vi "Initialise.vi"(8 "error in":errorcluster, 9 "Radial Points":i32) -> (0 "error out":errorcluster, 3 "Model Data":T2 {"Matricies"."K" format="%#_6e"; "Matricies"."Dout" format="%#_6e"; "Matricies"."Bout" format="%#_6e"; "Matricies"."Aout" format="%#_6e"; "Matricies"."Dint" format="%#_6e"; "Matricies"."Bint" format="%#_6e"; "Matricies"."Aint" format="%#_6e"; "Constants"."Z" format="%^#_6e"})   [LabVIEW 2012]
uses:
  Model Data.ctl
  PZT type.ctl
  Piezo_Discs.ctl
  LEM_Params.ctl
  Layer Properties.ctl
  Matricies.ctl
  <vilib>/Utility/error.llb/DialogType.ctl
  <vilib>/Analysis/1siggen.llb/Ramp Pattern by Samples.vi
  <vilib>/Analysis/NI_AALBase.lvlib
panel:
  out "Layer Properties":T1[](array[typedef])
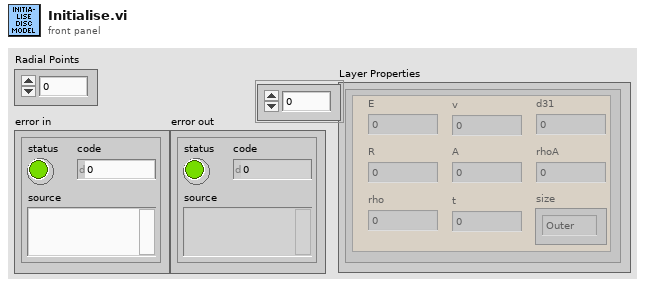
[diagram p1: front panel]
types:
  T1 = typedef "Layer Properties.ctl" = cluster{"E":dbl, "R":dbl, "rho":dbl, "rhoA":dbl, "v":dbl, "A":dbl, "t":dbl, "d31":dbl, "size":enum16{"Outer", "Inner"}}
  T2 = typedef "Model Data.ctl" = cluster{"Disc Properties":cluster{"Type":T3, "Disc Model":T4}, "Constants":cluster{"Radius":dbl[], "U(r)":dbl[], "W(r)":dbl[], "Vac":dbl, "P":dbl, "RiRo":dbl, "Area Density (r)":dbl[], "Ro":dbl, "Ri":dbl, "Z":dbl[], "Nr":dbl, "Mr":dbl, "c":dbl[], "AoC":dbl, "BoC":dbl, "AiC":dbl, "BiC":dbl, "f1":dbl, "f2":dbl}, "LEM Parameters":T5, "Layer Properties":T1[], "Matricies":T6}
  T3 = typedef "PZT type.ctl" = enum16{"Bimorph", "Unimorph"}
  T4 = typedef "Piezo_Discs.ctl" = enum16{"FTBD-21T-4.0A1", "PZT-5A (Gallas 1)", "PZT-5A (Gallas 2)", "AB4113B", "Create new disc...", "Load disc from file..."}
  T5 = typedef "LEM_Params.ctl" = cluster{"Displacement Ratio":dbl, "Cd":dbl, "Md":dbl, "xdc":dbl, "fd":dbl, "Sensitivity":dbl, "dA":dbl, "Rd":dbl, "Zeta":dbl, "Phi":dbl}
  T6 = typedef "Matricies.ctl" = cluster{"Aint":dbl[][], "Bint":dbl[][], "Dint":dbl[][], "Aout":dbl[][], "Bout":dbl[][], "Dout":dbl[][], "b":dbl[], "K":dbl[][]}
  T7 = typedef "DialogType.ctl" = u16
  T8 = typedef "Custom_Piezo.ctl" = cluster{"Young's Modulus":dbl, "Radius":dbl, "Density":dbl, "Poissoin's Ratio":dbl, "Thickness":dbl, "Dielectric Strength (d31)":dbl, "Type":T3}
  T9 = cluster{"Radius":dbl[], "U(r)":dbl[], "W(r)":dbl[], "Vac":dbl, "P":dbl, "RiRo":dbl, "Area Density (r)":dbl[], "Ro":dbl, "Ri":dbl, "Z":dbl[], "Nr":dbl, "Mr":dbl, "c":dbl[], "AoC":dbl, "BoC":dbl, "AiC":dbl, "BiC":dbl, "f1":dbl, "f2":dbl}
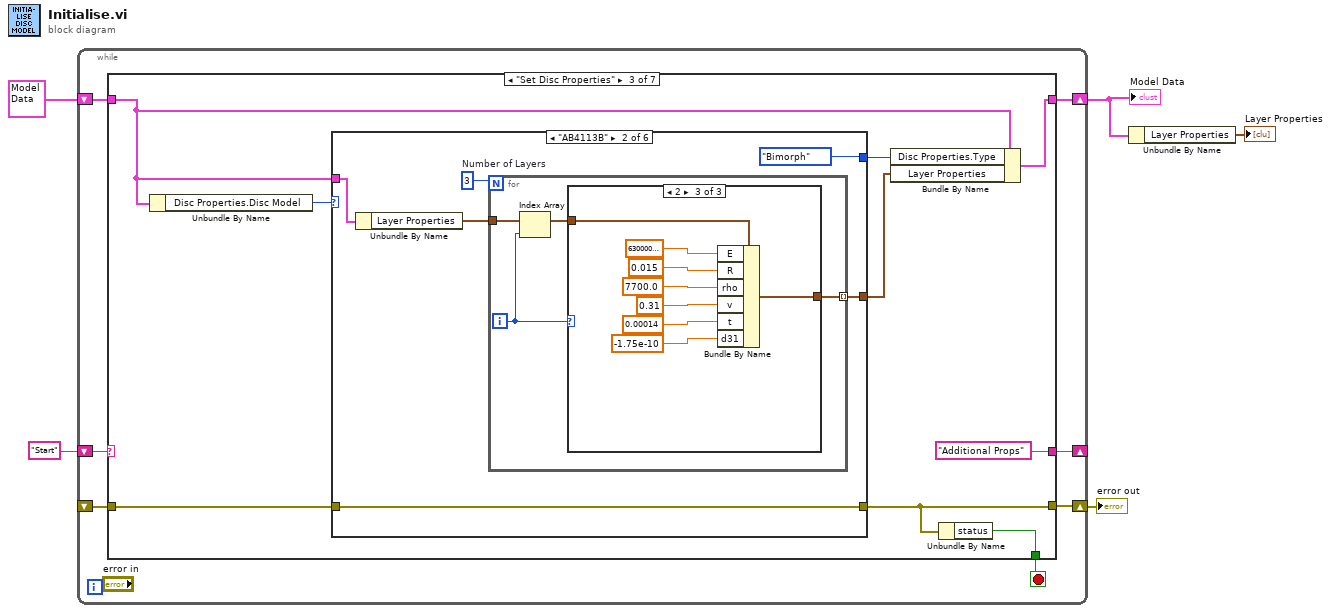
[diagram p0: block diagram]
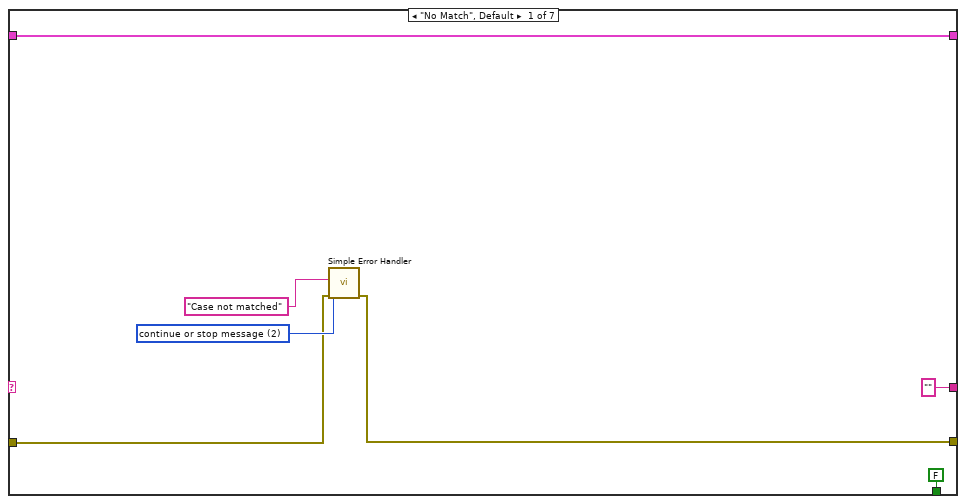
[diagram p2: hidden frame]
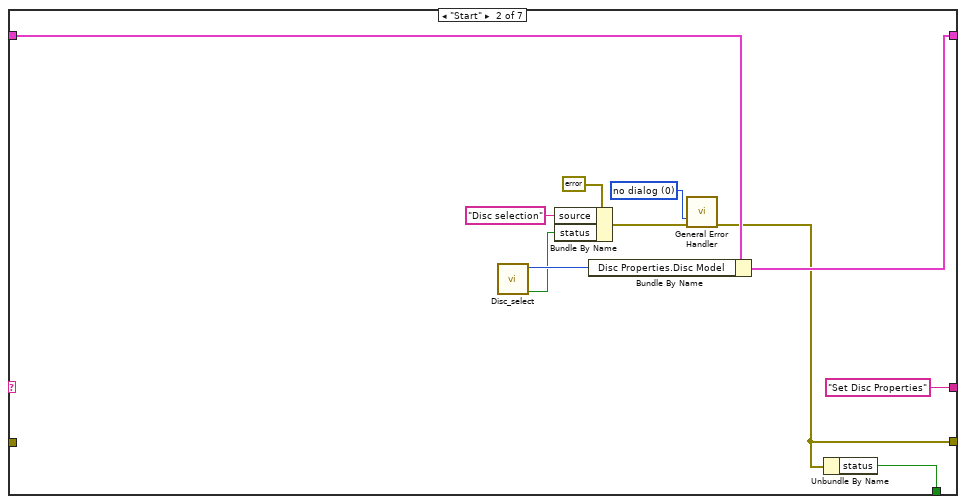
[diagram p3: hidden frame]
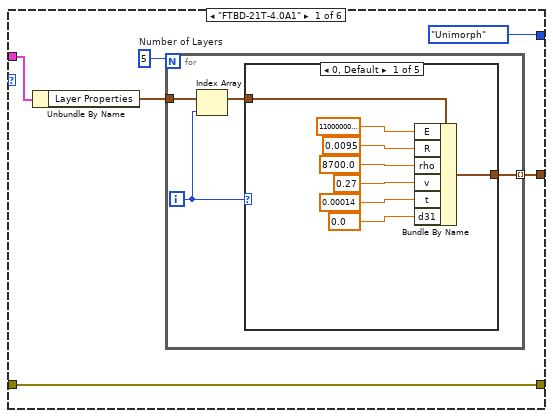
[diagram p4: hidden frame]
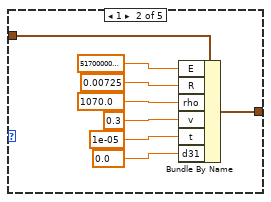
[diagram p5: hidden frame]
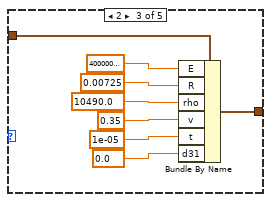
[diagram p6: hidden frame]
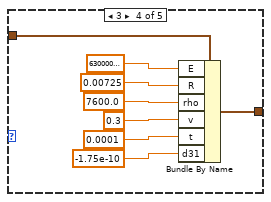
[diagram p7: hidden frame]
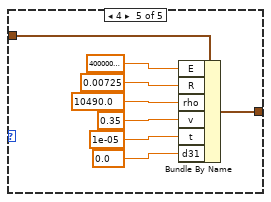
[diagram p8: hidden frame]
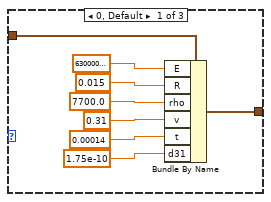
[diagram p9: hidden frame]
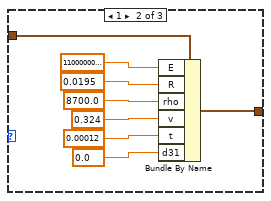
[diagram p10: hidden frame]
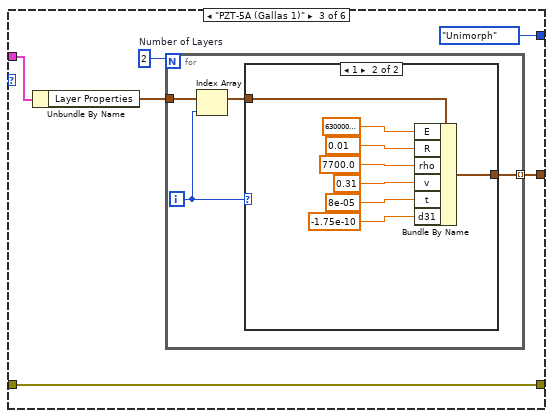
[diagram p11: hidden frame]
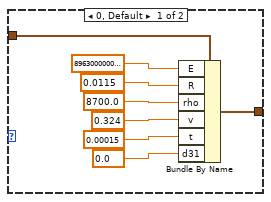
[diagram p12: hidden frame]
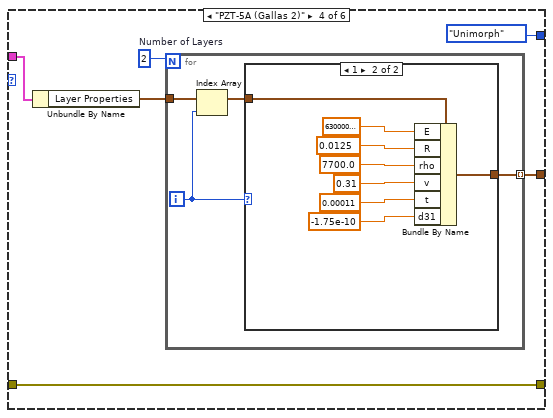
[diagram p13: hidden frame]
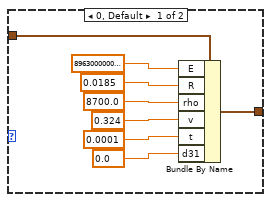
[diagram p14: hidden frame]
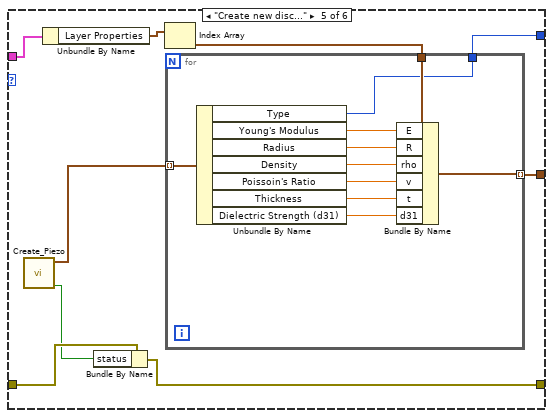
[diagram p15: hidden frame]
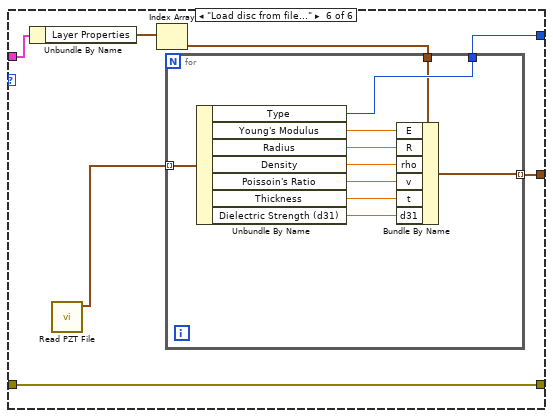
[diagram p16: hidden frame]
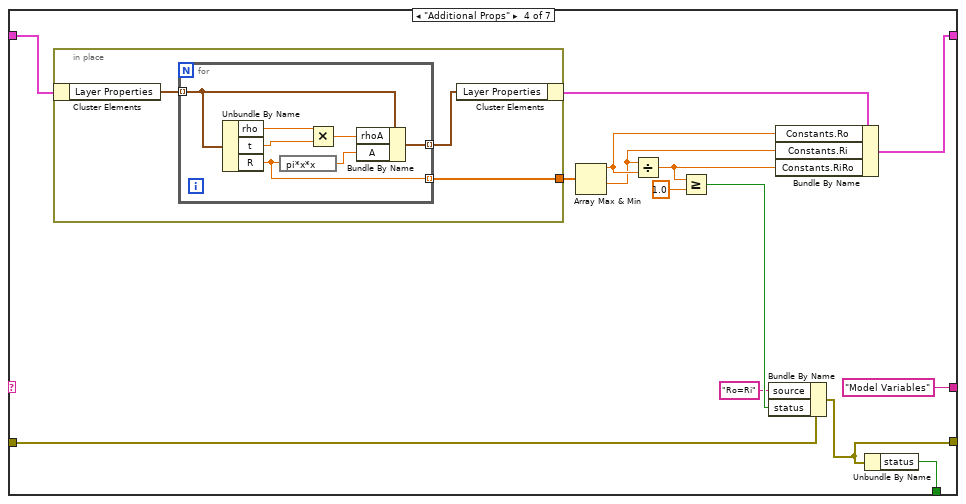
[diagram p17: hidden frame]
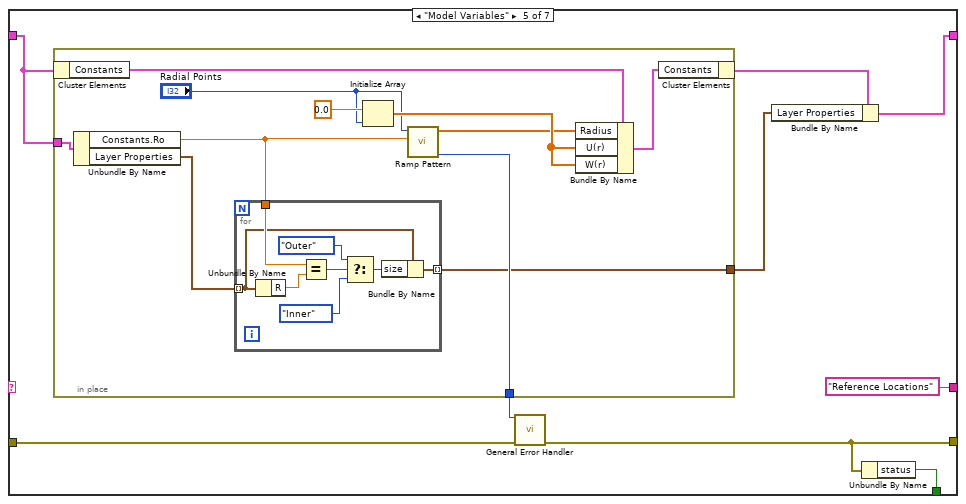
[diagram p18: hidden frame]
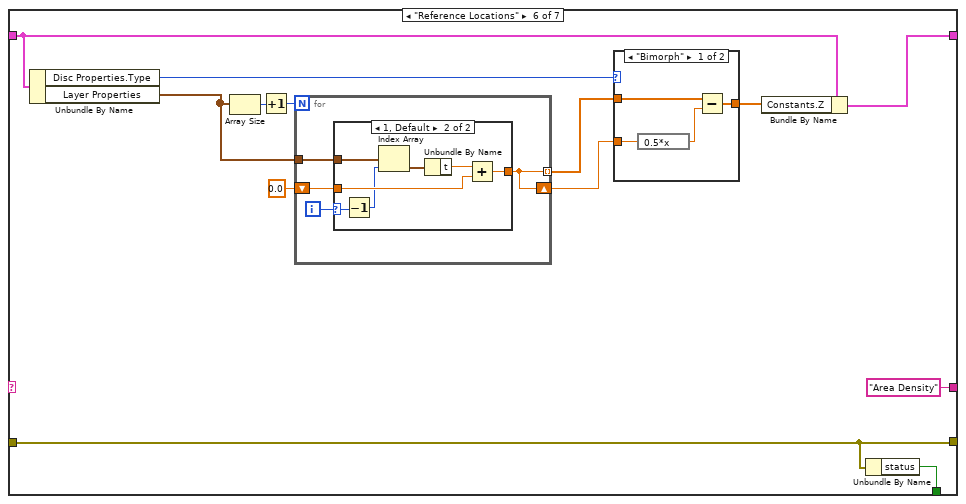
[diagram p19: hidden frame]
diagram:
  n1 = while {
    shift-right: [w10] -> _
    shift-left: "Start" -> [w11]
    shift-right: [w8] -> w2
    shift-left: T2 {"Disc Properties"={"Type"=enum."Bimorph", "Disc Model"=enum."FTBD-21T-4.0A1"}, "Constants"={"Radius"=[], "U(r)"=[], "W(r)"=[], "Vac"=0.0, "P"=0.0, "RiRo"=0.0, "Area Density (r)"=[], "Ro"=0.0, "Ri"=0.0, "Z"=[], "Nr"=0.0, "Mr"=0.0, "c"=[], "AoC"=0.0, "BoC"=0.0, "AiC"=0.0, "BiC"=0.0, "f1"=0.0, "f2"=0.0}, "LEM Parameters"={"Displacement Ratio"=0.0, "Cd"=0.0, "Md"=0.0, "xdc"=0.0, "fd"=0.0, "Sensitivity"=0.0, "dA"=0.0, "Rd"=0.0, "Zeta"=0.0, "Phi"=0.0}, "Layer Properties"=[], "Matricies"={"Aint"=[], "Bint"=[], "Dint"=[], "Aout"=[], "Bout"=[], "Dout"=[], "b"=[], "K"=[]}} ("Model Data") -> [w9]
    shift-right: [w7] -> w4
    shift-left: _ -> [w6]
    stop <- w12 stop-if-true
    n2 = case shown="\"Set Disc Properties\"" w11 {
      tunnel: [FALSE w20 w33 w218 w237 w264 TRUE] -> w12
      tunnel: ["" "Set Disc Properties" "Additional Props" "Model Variables" "Reference Locations" "Area Density" ""] -> w10
      tunnel: w9 -> [w18 w30 w37 w224 w244 w274 w299]
      tunnel: [w18 w28 w35 w219 w240 w273 w298] -> w8
      tunnel: [w13 w21 w32 w212 w236 w265 w306] -> w7
      tunnel: w6 -> [w14 _ w31 w215 w243 w265 w306]
      frame "No Match", Default {
        w15 = T7 2 items=["no dialog", "OK message", "continue or stop message", "OK message + warnings", "continue/stop + warnings"] ("type of dialog (OK msg:1)")
        n3 = call <vilib>:"Simple Error Handler.vi"("error source (\" \")"="Case not matched", "type of dialog (OK msg:1)"=w15, "error in (no error)"=w14) -> ("error out"=w13:errorcluster)  [unwired: 2 in, 4 out]
      }
      frame "Start" {
        w22 = T7 0 items=["no dialog", "OK message", "continue or stop message", "OK message + warnings", "continue/stop + warnings"] ("type of dialog (OK msg:1)")
        n4 = call "Disc_select.vi"() -> ("Cancel Button 2"=w24:bool, "Enum 2"=w29:T4)  [unwired: 10 in]
        n5 = Bundle By Name(cluster=errorcluster {"status"=FALSE, "code"=0, "source"=""} ("error constant"), "source"="Disc selection", "status"=w24) -> (w25:errorcluster)
        n6 = Bundle By Name(cluster=w30, "Disc Properties.Disc Model"=w29) -> (w28:T2)
        n7 = call <vilib>:"General Error Handler.vi"("type of dialog (OK msg:1)"=w22, "error in (no error)"=w25) -> ("error out"=w21:errorcluster)  [unwired: 9 in, 4 out]
        n8 = Unbundle By Name(w21) -> ("status"=w20:bool)
      }
      frame "Set Disc Properties" {
        n9 = Unbundle By Name(w37) -> ("Disc Properties.Disc Model"=w38:T4)
        n10 = case shown="\"AB4113B\"" w38 {
          tunnel: w37 -> [w44 w94 w128 w154 w184 w201]
          tunnel: [PZT_type."Unimorph" ("Type") PZT_type."Bimorph" ("Type") PZT_type."Unimorph" ("Type") PZT_type."Unimorph" ("Type") w178 w199] -> w36
          tunnel: [w42 w92 w126 w152 w183 w200] -> w34
          tunnel: [w41 w91 w125 w151 w179 w197] -> w32
          tunnel: w31 -> [w41 w91 w125 w151 w181 w197]
          frame "FTBD-21T-4.0A1" {
            w45 = 5  # Number of Layers
            n11 = Unbundle By Name(w44) -> ("Layer Properties"=w43:T1[])
            n12 = for {
              N: w45 -> [_]
              tunnel: w43 -> [w49]
              tunnel: [w48] -> w42 mode=indexing
              i -> [w46]
              n13 = Index Array(array=w49, index=w46) -> (element=w47:T1)
              n14 = case shown="0, Default" w46 {
                tunnel: w47 -> [w57 w65 w73 w81 w89]
                tunnel: [w56 w64 w72 w80 w88] -> w48
                frame 0, Default {
                  n15 = Bundle By Name(cluster=w57, "E"=110000000000.0, "R"=0.0095 ("E"), "rho"=8700.0 ("E"), "v"=0.27 ("E"), "t"=0.00014 ("E"), "d31"=0.0 ("E")) -> (w56:T1)
                }
                frame 1 {
                  n16 = Bundle By Name(cluster=w65, "E"=5170000000.0, "R"=0.00725 ("E"), "rho"=1070.0 ("E"), "v"=0.3 ("E"), "t"=1e-05 ("E"), "d31"=0.0 ("E")) -> (w64:T1)
                }
                frame 2 {
                  n17 = Bundle By Name(cluster=w73, "E"=40000000000.0, "R"=0.00725 ("E"), "rho"=10490.0 ("E"), "v"=0.35 ("E"), "t"=1e-05 ("E"), "d31"=0.0 ("E")) -> (w72:T1)
                }
                frame 3 {
                  n18 = Bundle By Name(cluster=w81, "E"=63000000000.0, "R"=0.00725 ("E"), "rho"=7600.0 ("E"), "v"=0.3 ("E"), "t"=0.0001 ("E"), "d31"=-1.75e-10 ("E")) -> (w80:T1)
                }
                frame 4 {
                  n19 = Bundle By Name(cluster=w89, "E"=40000000000.0, "R"=0.00725 ("E"), "rho"=10490.0 ("E"), "v"=0.35 ("E"), "t"=1e-05 ("E"), "d31"=0.0 ("E")) -> (w88:T1)
                }
              }
            }
          }
          frame "AB4113B" {
            w95 = 3  # Number of Layers
            n20 = Unbundle By Name(w94) -> ("Layer Properties"=w93:T1[])
            n21 = for {
              N: w95 -> [_]
              tunnel: w93 -> [w99]
              tunnel: [w98] -> w92 mode=indexing
              i -> [w96]
              n22 = Index Array(array=w99, index=w96) -> (element=w97:T1)
              n23 = case shown="2" w96 {
                tunnel: w97 -> [w101 w108 w116]
                tunnel: [w100 w109 w117] -> w98
                frame 0, Default {
                  n24 = Bundle By Name(cluster=w101, "E"=63000000000.0, "R"=0.015 ("E"), "rho"=7700.0 ("E"), "v"=0.31 ("E"), "t"=0.00014 ("E"), "d31"=1.75e-10 ("E")) -> (w100:T1)
                }
                frame 1 {
                  n25 = Bundle By Name(cluster=w108, "E"=110000000000.0, "R"=0.0195 ("E"), "rho"=8700.0 ("E"), "v"=0.324 ("E"), "t"=0.00012 ("E"), "d31"=0.0 ("E")) -> (w109:T1)
                }
                frame 2 {
                  n26 = Bundle By Name(cluster=w116, "E"=63000000000.0, "R"=0.015 ("E"), "rho"=7700.0 ("E"), "v"=0.31 ("E"), "t"=0.00014 ("E"), "d31"=-1.75e-10 ("E")) -> (w117:T1)
                }
              }
            }
          }
          frame "PZT-5A (Gallas 1)" {
            w129 = 2  # Number of Layers
            n27 = Unbundle By Name(w128) -> ("Layer Properties"=w127:T1[])
            n28 = for {
              N: w129 -> [_]
              tunnel: w127 -> [w133]
              tunnel: [w132] -> w126 mode=indexing
              i -> [w130]
              n29 = Index Array(array=w133, index=w130) -> (element=w131:T1)
              n30 = case shown="1" w130 {
                tunnel: w131 -> [w141 w149]
                tunnel: [w140 w148] -> w132
                frame 0, Default {
                  n31 = Bundle By Name(cluster=w141, "E"=89630000000.0, "R"=0.0115 ("E"), "rho"=8700.0 ("E"), "v"=0.324 ("E"), "t"=0.00015 ("E"), "d31"=0.0 ("E")) -> (w140:T1)
                }
                frame 1 {
                  n32 = Bundle By Name(cluster=w149, "E"=63000000000.0, "R"=0.01 ("E"), "rho"=7700.0 ("E"), "v"=0.31 ("E"), "t"=8e-05 ("E"), "d31"=-1.75e-10 ("E")) -> (w148:T1)
                }
              }
            }
          }
          frame "PZT-5A (Gallas 2)" {
            w155 = 2  # Number of Layers
            n33 = Unbundle By Name(w154) -> ("Layer Properties"=w153:T1[])
            n34 = for {
              N: w155 -> [_]
              tunnel: w153 -> [w159]
              tunnel: [w158] -> w152 mode=indexing
              i -> [w156]
              n35 = Index Array(array=w159, index=w156) -> (element=w157:T1)
              n36 = case shown="1" w156 {
                tunnel: w157 -> [w167 w175]
                tunnel: [w166 w174] -> w158
                frame 0, Default {
                  n37 = Bundle By Name(cluster=w167, "E"=89630000000.0, "R"=0.0185 ("E"), "rho"=8700.0 ("E"), "v"=0.324 ("E"), "t"=0.0001 ("E"), "d31"=0.0 ("E")) -> (w166:T1)
                }
                frame 1 {
                  n38 = Bundle By Name(cluster=w175, "E"=63000000000.0, "R"=0.0125 ("E"), "rho"=7700.0 ("E"), "v"=0.31 ("E"), "t"=0.00011 ("E"), "d31"=-1.75e-10 ("E")) -> (w174:T1)
                }
              }
            }
          }
          frame "Create new disc..." {
            n39 = call "Create_Piezo.vi"() -> ("Cancel Button Out"=w180:bool, "Layer Data Out"=w182:T8[])  [unwired: 10 in]
            n40 = Unbundle By Name(w184) -> ("Layer Properties"=w177:T1[])
            n41 = Bundle By Name(cluster=w181, "status"=w180) -> (w179:errorcluster)
            n42 = Index Array(array=w177) -> (element=w176:T1)  [unwired: 1 in]
            n43 = for {
              tunnel: w182 -> [w193] mode=indexing
              tunnel: [w185] -> w183 mode=indexing
              tunnel: w176 -> [w194]
              tunnel: [w192] -> w178
              n44 = Unbundle By Name(w193) -> ("Type"=w192:T3, "Young's Modulus"=w191:dbl, "Radius"=w190:dbl, "Density"=w189:dbl, "Poissoin's Ratio"=w188:dbl, "Thickness"=w187:dbl, "Dielectric Strength (d31)"=w186:dbl)
              n45 = Bundle By Name(cluster=w194, "E"=w191, "R"=w190, "rho"=w189, "v"=w188, "t"=w187, "d31"=w186) -> (w185:T1)
            }
          }
          frame "Load disc from file..." {
            n46 = Unbundle By Name(w201) -> ("Layer Properties"=w196:T1[])
            n47 = call "Read PZT File.vi"() -> ("Layers"=w198:T8[])  [unwired: 11 in]
            n48 = Index Array(array=w196) -> (element=w195:T1)  [unwired: 1 in]
            n49 = for {
              tunnel: w198 -> [w211] mode=indexing
              tunnel: [w203] -> w200 mode=indexing
              tunnel: [w210] -> w199
              tunnel: w195 -> [w202]
              n50 = Unbundle By Name(w211) -> ("Type"=w210:T3, "Young's Modulus"=w209:dbl, "Radius"=w208:dbl, "Density"=w207:dbl, "Poissoin's Ratio"=w206:dbl, "Thickness"=w205:dbl, "Dielectric Strength (d31)"=w204:dbl)
              n51 = Bundle By Name(cluster=w202, "E"=w209, "R"=w208, "rho"=w207, "v"=w206, "t"=w205, "d31"=w204) -> (w203:T1)
            }
          }
        }
        n52 = Bundle By Name(cluster=w37, "Disc Properties.Type"=w36, "Layer Properties"=w34) -> (w35:T2)
        n53 = Unbundle By Name(w32) -> ("status"=w33:bool)
      }
      frame "Additional Props" {
        n54 = in-place {
          in-place-border: [w226] -> w222
          n55 = in-place-cluster #1(w224) -> ("Layer Properties"=w228:T1[])
          n56 = for {
            tunnel: w228 -> [w231] mode=indexing
            tunnel: [w230] -> w226 mode=indexing
            tunnel: [w229] -> w227 mode=indexing
            n57 = Unbundle By Name(w231) -> ("rho"=w235:dbl, "t"=w232:dbl, "R"=w230:dbl)
            n58 = expression code="pi*x*x"(w230) -> (w233:dbl)
            n59 = Multiply(x=w235, y=w232) -> (x*y=w234:dbl)
            n60 = Bundle By Name(cluster=w231, "rhoA"=w234, "A"=w233) -> (w229:T1)
          }
          n61 = in-place-cluster #1("Layer Properties"=w227) -> (w223:T2)
        }
        n62 = Array Max & Min(array=w222) -> (max value=w221:dbl, min value=w220:dbl)  [unwired: 2 out]
        n63 = Divide(x=w220, y=w221) -> (x/y=w217:dbl)
        n64 = Greater Or Equal?(x=w217, y=1.0) -> (x >= y?=w214:bool)
        n65 = Bundle By Name(cluster=w215, "source"="Ro=Ri", "status"=w214) -> (w212:errorcluster)
        n66 = Bundle By Name(cluster=w223, "Constants.Ro"=w221, "Constants.Ri"=w220, "Constants.RiRo"=w217) -> (w219:T2)
        n67 = Unbundle By Name(w212) -> ("status"=w218:bool)
      }
      frame "Model Variables" {
        n68 = in-place {
          in-place-border: w244 -> [w251]
          in-place-border: [w249] -> w242
          in-place-border: [w245] -> w239
          n69 = in-place-cluster #2(w244) -> ("Constants"=w254:T9)
          n70 = Unbundle By Name(w251) -> ("Constants.Ro"=w247:dbl, "Layer Properties"=w248:T1[])
          n71 = for {
            tunnel: w247 -> [w262]
            tunnel: w248 -> [w258] mode=indexing
            tunnel: [w256] -> w245 mode=indexing
            n72 = Unbundle By Name(w258) -> ("R"=w263:dbl)
            n73 = Equal?(x=w262, y=w263) -> (x = y?=w261:bool)
            n74 = Select(t=enum16{"Outer", "Inner"}."Outer" ("size"), s=w261, f=enum16{"Outer", "Inner"}."Inner" ("size")) -> (s? t:f=w257:enum16{"Outer", "Inner"})
            n75 = Bundle By Name(cluster=w258, "size"=w257) -> (w256:T1)
          }
          n76 = Initialize Array(0.0 ("element"), "Radial Points") -> (w252:dbl[])
          n77 = call-poly <vilib>:"Ramp Pattern.vi"("end"=w247, "samples"="Radial Points") -> ("error"=w249:i32, "Ramp Pattern"=w250:dbl[])  [unwired: 8 in]
          n78 = Bundle By Name(cluster=w254, "Radius"=w250, "U(r)"=w252, "W(r)"=w252) -> (w253:T9)
          n79 = in-place-cluster #2("Constants"=w253) -> (w241:T2)
        }
        n80 = call <vilib>:"General Error Handler.vi"("[error code] (0)"=w242, "error in (no error)"=w243) -> ("error out"=w236:errorcluster)  [unwired: 9 in, 4 out]
        n81 = Bundle By Name(cluster=w241, "Layer Properties"=w239) -> (w240:T2)
        n82 = Unbundle By Name(w236) -> ("status"=w237:bool)
      }
      frame "Reference Locations" {
        n83 = Unbundle By Name(w274) -> ("Disc Properties.Type"=w269:T3, "Layer Properties"=w275:T1[])
        n84 = Array Size(array=w275) -> (size(s)=w272:i32)
        n85 = Increment(x=w272) -> (x+1=w271:i32)
        n86 = for {
          N: w271 -> [_]
          tunnel: w275 -> [w282]
          shift-right: [w283] -> w267
          shift-left: 0.0 ("t") -> [w284]
          tunnel: [w283] -> w268 mode=indexing
          i -> [w285]
          n87 = case shown="1, Default" w285 {
            selector: w285 -> [w288 w292]
            tunnel: [w290 w296] -> w283
            tunnel: w284 -> [_ w297]
            tunnel: w282 -> [w289 w294]
            frame 0 {
              n88 = Index Array(array=w289, index=w288) -> (element=w287:T1)
              n89 = Unbundle By Name(w287) -> ("t"=w286:dbl)
              n90 = expression code="-0.5*x"(w286) -> (w290:dbl)
            }
            frame 1, Default {
              n91 = Decrement(x=w292) -> (x-1=w291:i32)
              n92 = Index Array(array=w294, index=w291) -> (element=w295:T1)
              n93 = Unbundle By Name(w295) -> ("t"=w293:dbl)
              n94 = Add(x=w293, y=w297) -> (x+y=w296:dbl)
            }
          }
        }
        n95 = case shown="\"Bimorph\"" w269 {
          tunnel: w268 -> [w280 w281]
          tunnel: w267 -> [w279 _]
          tunnel: [w278 w281] -> w266
          frame "Bimorph" {
            n96 = expression code="0.5*x"(w279) -> (w277:dbl)
            n97 = Subtract(x=w280, y=w277) -> (x-y=w278:dbl[])
          }
          frame "Unimorph" {
          }
        }
        n98 = Bundle By Name(cluster=w274, "Constants.Z"=w266) -> (w273:T2)
        n99 = Unbundle By Name(w265) -> ("status"=w264:bool)
      }
      frame "Area Density" {
        n100 = Unbundle By Name(w299) -> ("Constants.Radius"=w304:dbl[], "Layer Properties"=w303:T1[])
        n101 = for {
          tunnel: w304 -> [w312]
          tunnel: w303 -> [w311] mode=indexing
          tunnel: [w310] -> w302 mode=indexing
          n102 = for {
            tunnel: w312 -> [w319] mode=indexing
            tunnel: w311 -> [w318]
            tunnel: [w313] -> w310 mode=indexing
            n103 = Unbundle By Name(w318) -> ("rhoA"=w314:dbl, "R"=w317:dbl)
            n104 = Less?(x=w319, y=w317) -> (x < y?=w316:bool)
            n105 = Select(t=w314, s=w316, f=0.0) -> (s? t:f=w313:dbl)
          }
        }
        n106 = Transpose 2D Array(2D array=w302) -> (transposed array=w301:dbl[][])
        n107 = for {
          tunnel: w301 -> [w309] mode=indexing
          tunnel: [w308] -> w300 mode=indexing
          n108 = Add Array Elements(numeric array=w309) -> (sum=w308:dbl)
        }
        n109 = Bundle By Name(cluster=w299, "Constants.Area Density (r)"=w300) -> (w298:T2)
      }
    }
  }
  "error out" <- w4
  "Model Data" <- w2
  n110 = Unbundle By Name(w2) -> ("Layer Properties"=→"Layer Properties":T1[])
